vi "ProdaNG.Tree.Release.GetAll.vi"(7 "TestStepsTree":refnum<vi>, 8 "error in (no error)":errorcluster, 9 "Release":bool) -> (0 "error out":errorcluster, 2 "Elements to release":T1[](array[typedef]))   [LabVIEW 2016]
uses:
  ProdaNG.Tree.Fglb.Data.ctl
  ProdaNG.Tree.Fglb.Element.ctl
  ProdaNG.Tree.Fglb.Action.ctl
  ProdaNG.Configurator.Glb.vi
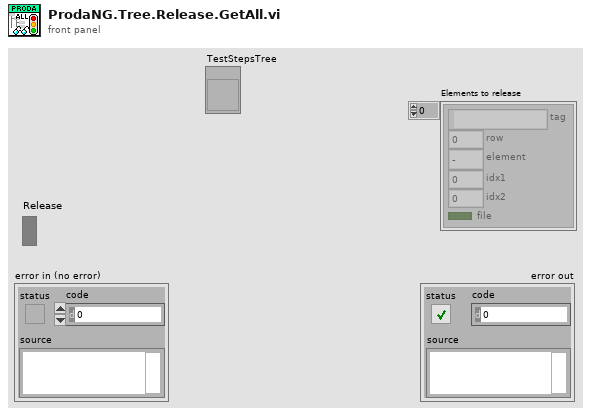
[diagram p1: front panel]
types:
  T1 = typedef "ProdaNG.Tree.Fglb.Data.ctl" = cluster{"tag":string, "row":i32, "element":T2, "idx1":i32, "idx2":i32, "file":bool}
  T2 = typedef "ProdaNG.Tree.Fglb.Element.ctl" = enum16{"-", "PP", "TS", "TP", "TV"}
  T3 = typedef "ProdaNG.Tree.Fglb.Action.ctl" = enum16{"init", "add", "get by row", "get by tag", "get by idx"}
  T4 = typedef "ProdaNG.TestStep.ctl" = cluster{"i_id":i32, "processStepId":i32, "testSequence":i32, "testOrder":i32, "mdReason":string, "mdUser":string, "mdTime":string, "description":string}
  T5 = typedef "ProdaNG.TestStepParam.ctl" = cluster{"i_id":i32, "testStepId":i32, "unitId":i32, "contentId":string, "previewId":string, "value":dbl, "valueText":string, "paramSequence":i32, "history":i32, "mdReason":string, "mdUser":string, "mdTime":string, "description":string}
  T6 = typedef "ProdaNG.TestValue.ctl" = cluster{"i_id":i32, "testStepId":i32, "releaseId":i32, "unitId":i32, "contentId":string, "previewId":string, "maximum":dbl, "minimum":dbl, "valueText":string, "testValueSequence":i32, "history":i32, "mdReason":string, "mdUser":string, "mdTime":string, "description":string}
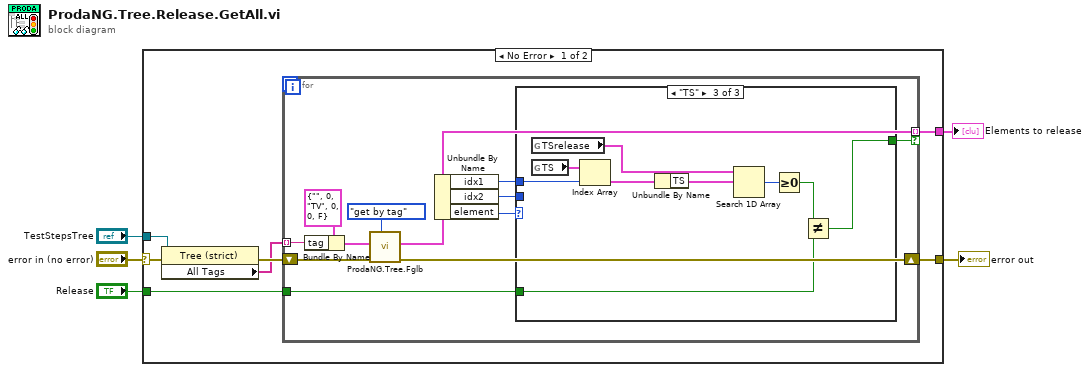
[diagram p0: block diagram]
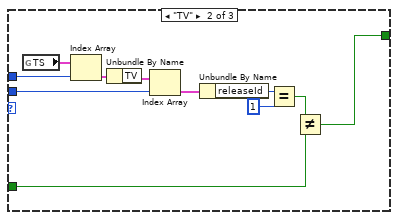
[diagram p3: hidden frame]
diagram:
  n1 = case shown="No Error" "error in (no error)" {
    selector: "error in (no error)" -> [w12 w45]
    tunnel: "TestStepsTree" -> [w9 _]
    tunnel: [w10 w45] -> w5
    tunnel: "Release" -> [w7 _]
    tunnel: [w6 _] -> w1
    frame No Error {
      n2 = property on="Property Node" class="Tree (strict)"(reference=w9, error in=w12) -> (error out=w11:errorcluster, "All Tags"=w8:string[])  [unwired: 1 out]
      n3 = for {
        tunnel: w8 -> [w21] mode=indexing
        shift-right: [w14] -> w10
        shift-left: w11 -> [w20]
        tunnel: w7 -> [w17]
        tunnel: [w16] -> w6 mode=indexing if=w15
        n4 = Bundle By Name(cluster=T1 {"tag"="", "row"=0, "element"=enum."TV", "idx1"=0, "idx2"=0, "file"=FALSE} ("entry in"), "tag"=w21) -> (w22:T1)
        n5 = call "ProdaNG.Tree.Fglb.vi"("Action (add)"=ProdaNG.Tree.Fglb.Action."get by tag", "error in"=w20, "entry in"=w22) -> ("error out"=w14:errorcluster, "found entry"=w16:T1)  [unwired: 6 in, 1 out]
        n6 = Unbundle By Name(w16) -> ("idx1"=w18:i32, "idx2"=w13:i32, "element"=w19:T2)
        n7 = case shown="\"TS\"" w19 {
          tunnel: w18 -> [_ w35 w43]
          tunnel: w17 -> [_ w29 w38]
          tunnel: [_ w28 w37] -> w15
          tunnel: w13 -> [_ w26 _]
          frame Default {
          }
          frame "TV" {
            n8 = global read "ProdaNG.Configurator.Glb.vi" "TS"() -> (w34:cluster{"TS":T4, "TP":T5[], "TV":T6[]}[])
            n9 = Index Array(array=w34, index=w35) -> (element=w33:cluster{"TS":T4, "TP":T5[], "TV":T6[]})
            n10 = Unbundle By Name(w33) -> ("TV"=w27:T6[])
            n11 = Index Array(array=w27, index=w26) -> (element=w25:T6)
            n12 = Unbundle By Name(w25) -> ("releaseId"=w32:i32)
            n13 = Equal?(x=w32, y=1) -> (x = y?=w30:bool)
            n14 = Not Equal?(x=w30, y=w29) -> (x != y?=w28:bool)
          }
          frame "TS" {
            n15 = global read "ProdaNG.Configurator.Glb.vi" "TSrelease"() -> (w41:T4[])
            n16 = global read "ProdaNG.Configurator.Glb.vi" "TS"() -> (w44:cluster{"TS":T4, "TP":T5[], "TV":T6[]}[])
            n17 = Index Array(array=w44, index=w43) -> (element=w42:cluster{"TS":T4, "TP":T5[], "TV":T6[]})
            n18 = Unbundle By Name(w42) -> ("TS"=w36:T4)
            n19 = Search 1D Array(1D array=w41, element=w36) -> (index of element=w40:i32)  [unwired: 1 in]
            n20 = Greater Or Equal To 0?(x=w40) -> (x >= 0?=w39:bool)
            n21 = Not Equal?(x=w39, y=w38) -> (x != y?=w37:bool)
          }
        }
      }
    }
    frame Error {
    }
  }
  "error out" <- w5
  "Elements to release" <- w1
